vi "ztscopeM Trigger.vi"(6 "Slope":i32(ring) items=["Rising Edge", "Falling Edge"], 7 "error in":errorcluster, 8 "Level":dbl, 9 "Trigger Source":i32(ring)=10 items=["TTL0", "TTL1", "TTL2", "TTL3", "TTL4", "TTL5", "TTL6", "TTL7", "ECL0", "ECL1", "Input Channel 1", "Input Channel 2", "Input Channel 3", "Input Channel 4", "External Trigger Source", "STAR", "Manual Trigger", "Pattern"], 10 "Instrument Handle In":i32) -> (0 "error out":errorcluster, 3 "Instrument Handle Out":i32)   [LabVIEW 2013]
doc: "Set the trigger to detect an edge trigger event and configure the edge trigger settings."
uses:
  ztscopeM.dll
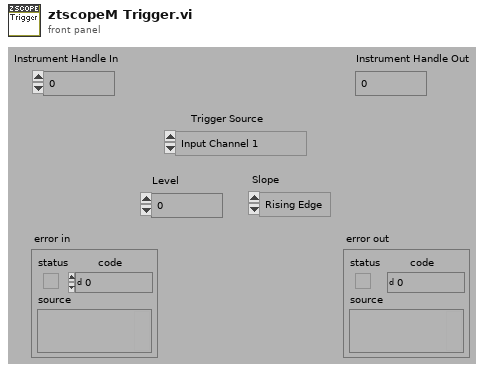
[diagram p1: front panel]
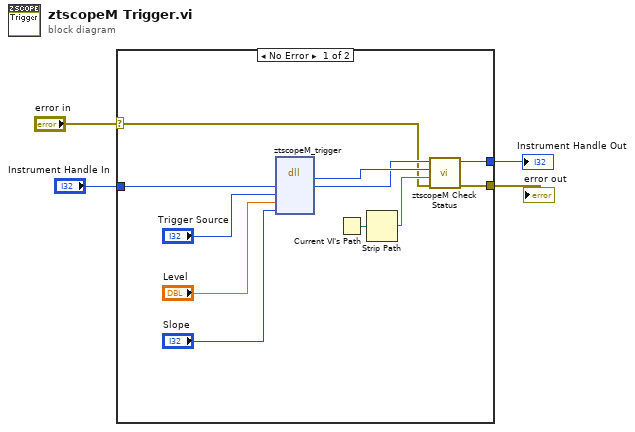
[diagram p0: block diagram]
diagram:
  n1 = case shown="No Error" "error in" {
    selector: "error in" -> [w7 w17]
    tunnel: [w6 w17] -> w1
    tunnel: "Instrument Handle In" -> [w15 w16]
    tunnel: [w5 w16] -> w3
    frame No Error {
      n2 = dll-call lib="C:/Program Files/National Instruments/instr.lib/ztscopem/ztscopeM.dll" fn="ztscopeM_trigger"("instrumentHandle"=w15, "triggerSource"="Trigger Source", "level"="Level", "slope"="Slope") -> (w9:i32, "instrumentHandle"=w8:i32)  [unwired: 6 in, 2 out]
      n3 = Current VI's Path() -> (path=w11:path)
      n4 = Strip Path(path=w11) -> (name=w10:string)  [unwired: 1 out]
      n5 = call "ztscopeM Check Status.vi"("error in"=w7, "name of VI"=w10, "status"=w9, "instrument handle in"=w8) -> ("error out"=w6:errorcluster, "instrument handle out"=w5:i32)  [unwired: 2 in]
    }
    frame Error {
    }
  }
  "Instrument Handle Out" <- w3
  "error out" <- w1
